vi "C to K (dbl).vi"(1 "C":dbl) -> (0 "K":dbl)   [LabVIEW 2012, in "Temp Converter.lvlib"]
doc: "<B>输入端子C</B>: 输入摄氏温度。\n<B>输出端子C</B>: 输出开氏温度。\n\n公式： K=C+273.15.\n创建者：CSXCS_366"
uses:
  Temp Converter.lvlib
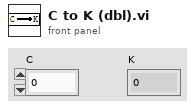
[diagram p1: front panel]
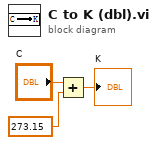
[diagram p0: block diagram]
diagram:
  n1 = Add(x="C", y=273.15) -> (x+y=→"K":dbl)
